vi "Parse Current Temperature.vi"(8 "Error In":errorcluster, 9 "Data":string, 10 "Device ID":string, 11 "Nest Config":T1) -> (0 "Error Out":errorcluster, 1 "Data":string, 2 "Current Temp":dbl, 3 "Nest Config":T1)   [LabVIEW 2013, in "LMH-Nest.lvlib"]
doc: "Get current temp."
uses:
  LMH-Nest.lvlib
  Type Defs/Nest Config.ctl
  <vilib>/httpClient/ClientHandle.ctl
  Type Defs/Session Data.ctl
  <vilib>/httpClient/LabVIEWHTTPClient.lvlib
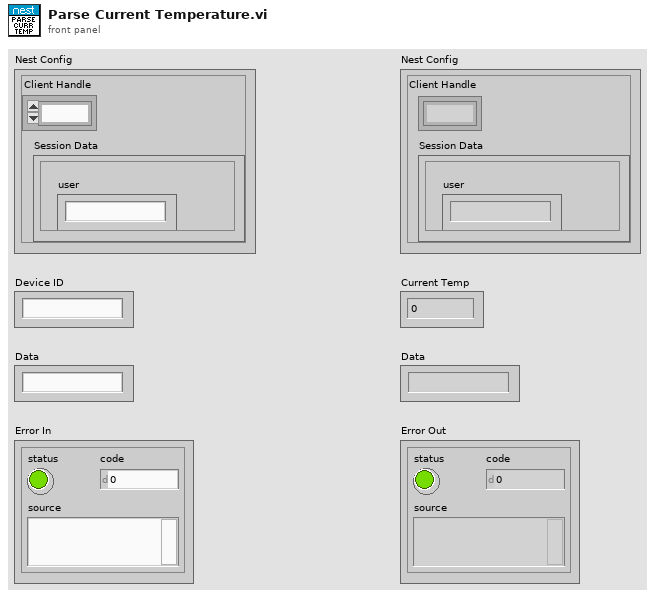
[diagram p1: front panel]
types:
  T1 = typedef "LMH-Nest.lvlib/Nest Config.ctl" = cluster{"Client Handle":T2, "Session Data":T3}
  T2 = typedef "LabVIEWHTTPClient.lvlib/ClientHandle.ctl" = refnum<k1>
  T3 = typedef "LMH-Nest.lvlib/Session Data.ctl" = cluster{"is_superuser":bool, "is_staff":bool, "urls":cluster{"transport_url":string, "rubyapi_url":string, "weather_url":string, "log_upload_url":string, "support_url":string}, "limits":cluster{"thermostats_per_structure":u32, "structures":u32, "thermostats":u32, "smoke_detectors":u32, "smoke_detectors_per_structure":u32}, "access_token":string, "userid":string, "expires_in":string, "email":string, "user":string, "language":string}
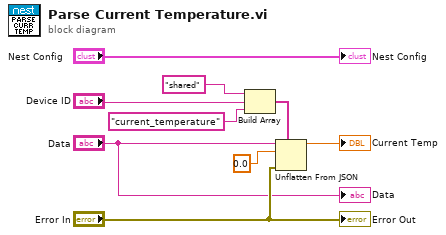
[diagram p0: block diagram]
diagram:
  n1 = Build Array("shared", "Device ID", "current_temperature" ("element")) -> (w7:string[])
  n2 = Unflatten From JSON(path=w7, JSON string="Data", type and defaults=0.0, error in (no error)="Error In") -> (value=→"Current Temp":dbl)  [unwired: 3 in, 1 out]
  "Nest Config" <- "Nest Config"
  "Error Out" <- "Error In"
  "Data" <- "Data"
